vi "IF2_UnixTimestamp.vi"() -> (3 "unixTimeStamp":u64)   [LabVIEW 2015, in "IF2_Reader.lvlib"]
uses:
  IF2_Reader.lvlib
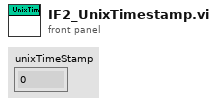
[diagram p1: front panel]
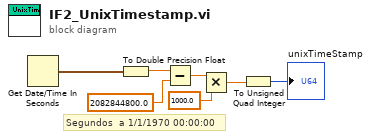
[diagram p0: block diagram]
diagram:
  # "Segundos  a 1/1/1970 00:00:00"
  n1 = Get Date/Time In Seconds() -> (seconds since 1Jan1904=w5:timestamp)
  n2 = To Double Precision Float(number=w5) -> (double precision float=w2:dbl)
  n3 = Subtract(x=w2, y=2082844800.0) -> (x-y=w3:dbl)
  n4 = Multiply(x=w3, y=1000.0) -> (x*y=w6:dbl)
  n5 = To Unsigned Quad Integer(1:w6) -> (0:→"unixTimeStamp":u64)
